vi "generate channels.vi"(10 "ch count":i32=10, 11 "TEC configuration in":refnum<class "TEC configuration.lvclass">) -> (0 "error out":errorcluster, 3 "TEC configuration out":refnum<class "TEC configuration.lvclass">)   [LabVIEW 2014, in "TEC tests.lvlib"]
uses:
  TEC tests.lvlib
  configuration/TEC configuration.lvclass
  <vilib>/NI/Tag Bus/tag/Data Type.ctl
  <vilib>/NI/Tag Bus Module Framework/channel/channel classification.ctl
  <vilib>/NI/Tag Bus/tag/tag descriptor.lvclass/tag descriptor.ctl
  <vilib>/NI/Tag Bus/tag/write raw default value.vi
  <vilib>/NI/Tag Bus/tag/tag descriptor.lvclass
  <vilib>/NI/Tag Bus Module Framework/channel/TBM channel.lvclass
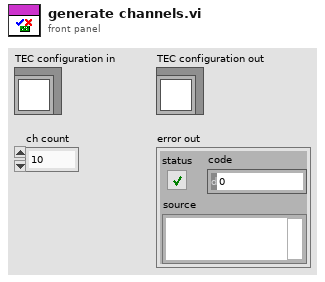
[diagram p1: front panel]
types:
  T1 = typedef "tag bus.lvlib/tag descriptor.lvclass/Data Type.ctl" = enum16{"Double", "Single", "I64", "I32", "I16", "I8", "U64", "U32", "U16", "U8", "Boolean", "String", "Array of Double", "Array of Single", "Array of I64", "Array of I32", "Array of I16", "Array of I8", "Array of U64", "Array of U32", "Array of U16", "Array of U8", "Array of Boolean", "Array of String"}
  T2 = typedef "TBM channel.lvclass/channel classification.ctl" = enum16{"input data", "output data", "processing parameter", "processing result"}
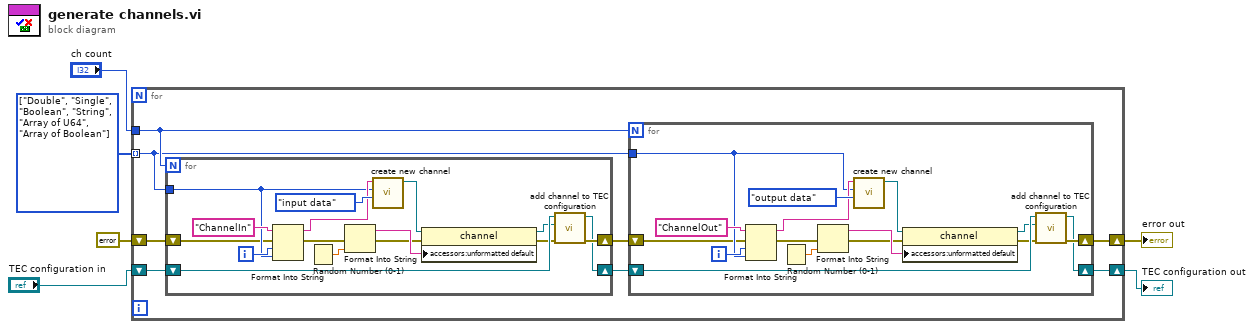
[diagram p0: block diagram]
diagram:
  w1 = T1[] [enum."Double", enum."Single", enum."Boolean", enum."String", enum."Array of U64", enum."Array of Boolean"] items=["Double", "Single", "I64", "I32", "I16", "I8", "U64", "U32", "U16", "U8", "Boolean", "String", "Array of Double", "Array of Single", "Array of I64", "Array of I32", "Array of I16", "Array of I8", "Array of U64", "Array of U32", "Array of U16", "Array of U8", "Array of Boolean", "Array of String"]
  n1 = for {
    tunnel: "ch count" -> [w13]
    shift-right: [w12] -> w4
    shift-left: "TEC configuration in" -> [w14]
    shift-right: [w9] -> w2
    shift-left: errorcluster {"status"=FALSE, "code"=0, "source"=""} ("error out") -> [w11]
    tunnel: w1 -> [w7] mode=indexing
    n2 = for {
      N: w13 -> [_]
      shift-right: [w25] -> w8
      shift-left: w14 -> [w24]
      shift-right: [w26] -> w10
      shift-left: w11 -> [w18]
      tunnel: w7 -> [w22]
      i -> [w29]
      n3 = Format Into String(initial string="ChannelIn" ("channel name"), error in=w18, w29, w22) -> (resulting string=w28:string, error out=w17:errorcluster)  [unwired: 1 in]
      n4 = Random Number (0-1)() -> (number: 0 to 1=w20:dbl)
      n5 = Format Into String(error in=w17, w20) -> (resulting string=w19:string, error out=w16:errorcluster)  [unwired: 2 in]
      n6 = call <vilib>:"create new channel.vi"("channel classification"=channel_classification."input data", "data type"=w22, "channel name"=w28) -> ("channel"=w23:refnum<class "TBM channel.lvclass">)  [unwired: 8 in]
      n7 = property class="channel"(reference=w23, error in=w16, "accessors:unformatted default"=w19) -> (reference out=w21:refnum<class "TBM channel.lvclass">, error out=w15:errorcluster)
      n8 = call "add channel to TEC configuration.vi"("error in"=w15, "channel"=w21, "TEC configuration in"=w24) -> ("error out"=w26:errorcluster, "TEC configuration out"=w25:refnum<class "TEC configuration.lvclass">)  [unwired: 7 in]
    }
    n9 = for {
      N: w13 -> [_]
      shift-right: [w40] -> w12
      shift-left: w8 -> [w42]
      shift-right: [w41] -> w9
      shift-left: w10 -> [w34]
      tunnel: w7 -> [w38]
      i -> [w45]
      n10 = Format Into String(initial string="ChannelOut" ("channel name"), error in=w34, w45, w38) -> (resulting string=w44:string, error out=w33:errorcluster)  [unwired: 1 in]
      n11 = Random Number (0-1)() -> (number: 0 to 1=w36:dbl)
      n12 = Format Into String(error in=w33, w36) -> (resulting string=w35:string, error out=w32:errorcluster)  [unwired: 2 in]
      n13 = call <vilib>:"create new channel.vi"("channel classification"=channel_classification."output data", "data type"=w38, "channel name"=w44) -> ("channel"=w39:refnum<class "TBM channel.lvclass">)  [unwired: 8 in]
      n14 = property class="channel"(reference=w39, error in=w32, "accessors:unformatted default"=w35) -> (reference out=w37:refnum<class "TBM channel.lvclass">, error out=w31:errorcluster)
      n15 = call "add channel to TEC configuration.vi"("error in"=w31, "channel"=w37, "TEC configuration in"=w42) -> ("error out"=w41:errorcluster, "TEC configuration out"=w40:refnum<class "TEC configuration.lvclass">)  [unwired: 7 in]
    }
  }
  "TEC configuration out" <- w4
  "error out" <- w2
